vi "Register.vi"(0 "BroadcastRegistry in":refnum<class "BroadcastRegistry.lvclass">, 5 "status":string="status", 7 "source":string="source", 9 "api":string="api", 11 "target":string="target") -> (4 "BroadcastRegistry out":refnum<class "BroadcastRegistry.lvclass">)   [LabVIEW 2020, in "Communicable State Machine.lvlib" / "BroadcastRegistry.lvclass"]
uses:
  BroadcastRegistry.lvclass
  BroadcastRegistry.lvclass/BroadcastRegistry.ctl
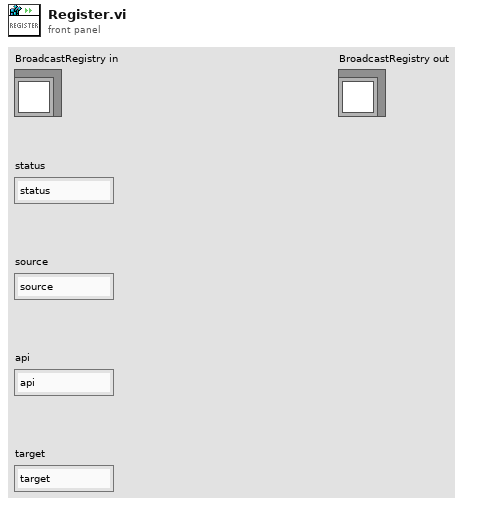
[diagram p1: front panel]
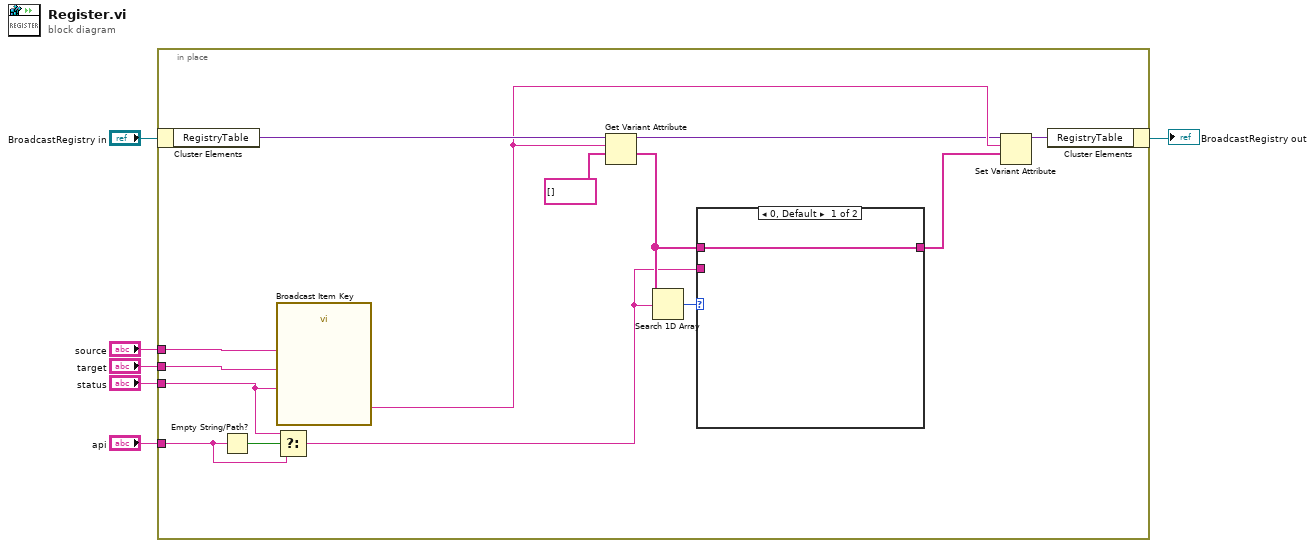
[diagram p0: block diagram]
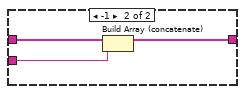
[diagram p2: hidden frame]
diagram:
  n1 = in-place {
    in-place-border: "status" -> [w19]
    in-place-border: "target" -> [w18]
    in-place-border: "source" -> [w17]
    in-place-border: "api" -> [w16]
    n2 = in-place-cluster #1("BroadcastRegistry in") -> ("RegistryTable"=w15:variant)
    n3 = Empty String/Path?(string/path=w16) -> (empty?=w20:bool)
    n4 = call "Broadcast Item Key.vi"("status"=w19, "target"=w18, "source"=w17) -> ("key"=w14:string)  [unwired: 2 in]
    n5 = Select(t=w19, s=w20, f=w16) -> (s? t:f=w7:string)
    n6 = Get Variant Attribute(Variant=w15, name=w14, default value (empty Variant)=string[] [] ("output cluster")) -> (duplicate Variant=w11:variant, value=w9:string[])  [unwired: 1 in, 2 out]
    n7 = Search 1D Array(1D array=w9, element=w7) -> (index of element=w12:i32)  [unwired: 1 in]
    n8 = case shown="0, Default" w12 {
      tunnel: w9 -> [w21 w24]
      tunnel: [w21 w23] -> w8
      tunnel: w7 -> [_ w22]
      frame 0, Default {
      }
      frame -1 {
        n9 = Build Array (concatenate)(w24, w22) -> (w23:string[])
      }
    }
    n10 = Set Variant Attribute(Variant=w11, name=w14, value=w8) -> (Variant out=w13:variant)  [unwired: 1 in, 2 out]
    n11 = in-place-cluster #1("RegistryTable"=w13) -> (→"BroadcastRegistry out":refnum<class "BroadcastRegistry.lvclass">)
  }
